vi "Shift U32 Number to get block exponent number.vi"(8 "Input Valid":bool=TRUE, 10 "Leading Zero Position":u8, 11 "Binary Number":u32 format="%.0b") -> (0 "Output Valid":bool=TRUE, 2 "Block Float Exponent":i8, 3 "Block Float Mantissa":u32)   [LabVIEW 2010]
uses:
  <vilib>/rvi/FXPMathLib/basic elements/FxpDiscreteDelay/XNode/nifxpmath_DiscreteDelay.xnode
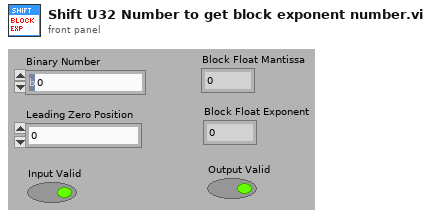
[diagram p1: front panel]
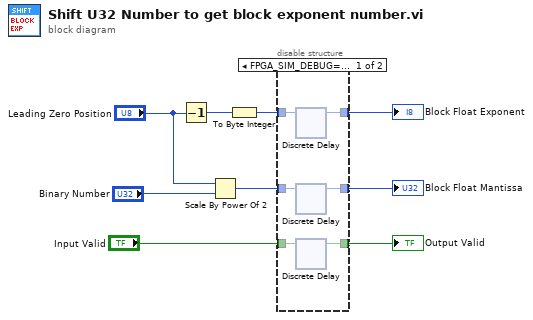
[diagram p0: block diagram]
diagram:
  n1 = Decrement(x="Leading Zero Position") -> (x-1=w9:u8)
  n2 = Scale By Power Of 2(n="Leading Zero Position", x="Binary Number") -> (x*2^n=w6:u32)
  n3 = To Byte Integer(number=w9) -> (8bit integer=w5:i8)
  n4 = disable-structure shown="FPGA_SIM_DEBUG==FALSE, default" {
    disable-tunnel: w6 -> [w15 w113]
    disable-tunnel: w5 -> [w14 w114]
    disable-tunnel: "Input Valid" -> [w13 w112]
    disable-tunnel: [w12 w114] -> w3
    disable-tunnel: [w11 w113] -> w2
    disable-tunnel: [w10 w112] -> w1
    frame condition #0 {
      n5 = xnode "Discrete Delay"("D"=w14) -> ("Q"=w12:i8)
      n6 = xnode "Discrete Delay"("D"=w15) -> ("Q"=w11:u32)
      n7 = xnode "Discrete Delay"("D"=w13) -> ("Q"=w10:bool)
    }
    frame condition #1 (active) {
    }
  }
  "Block Float Mantissa" <- w2
  "Block Float Exponent" <- w3
  "Output Valid" <- w1
